vi "PM5000_Power_demo.vi"(2 "error in (no error)":errorcluster) -> (0 "error out":errorcluster, 1 "Power Meter Out":T1)   [LabVIEW 2018]
panel:
  in  "Variacion Pontencia":sgl=0.1
  in  "Potencia Nominal":sgl=20.0
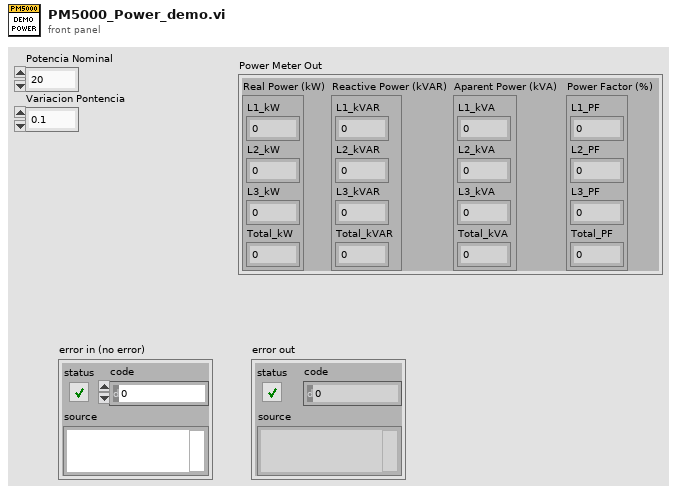
[diagram p1: front panel]
types:
  T1 = cluster{"Real Power (kW)":cluster{"L1_kW":sgl, "L2_kW":sgl, "L3_kW":sgl, "Total_kW":sgl}, "Reactive Power (kVAR)":cluster{"L1_kVAR":sgl, "L2_kVAR":sgl, "L3_kVAR":sgl, "Total_kVAR":sgl}, "Aparent Power (kVA)":cluster{"L1_kVA":sgl, "L2_kVA":sgl, "L3_kVA":sgl, "Total_kVA":sgl}, "Power Factor (%)":cluster{"L1_PF":sgl, "L2_PF":sgl, "L3_PF":sgl, "Total_PF":sgl}}
  T2 = cluster{"Real Power (kW)":cluster{"L1_kW":sgl, "L2_kW":sgl, "L3_kW":sgl, "Total_kW":sgl}, "Reactive Power (kVAR)":cluster{"L1_kVAR":sgl, "L2_kVAR":sgl, "L3_kVAR":sgl, "Total_kVAR":sgl}, "Aparent Power (kVA)":cluster{"L1_kVA":sgl, "L2_kVA":sgl, "L3_kVA":sgl, "Total_kVA":sgl}, "Power Factor":cluster{"L1_PF":sgl, "L2_PF":sgl, "L3_PF":sgl, "Total_PF":sgl}}
  T3 = cluster{"L1_PF":sgl, "L2_PF":sgl, "L3_PF":sgl, "Total_PF":sgl}
  T4 = cluster{"L1_kVA":sgl, "L2_kVA":sgl, "L3_kVA":sgl, "Total_kVA":sgl}
  T5 = cluster{"L1_kVAR":sgl, "L2_kVAR":sgl, "L3_kVAR":sgl, "Total_kVAR":sgl}
  T6 = cluster{"L1_kW":sgl, "L2_kW":sgl, "L3_kW":sgl, "Total_kW":sgl}
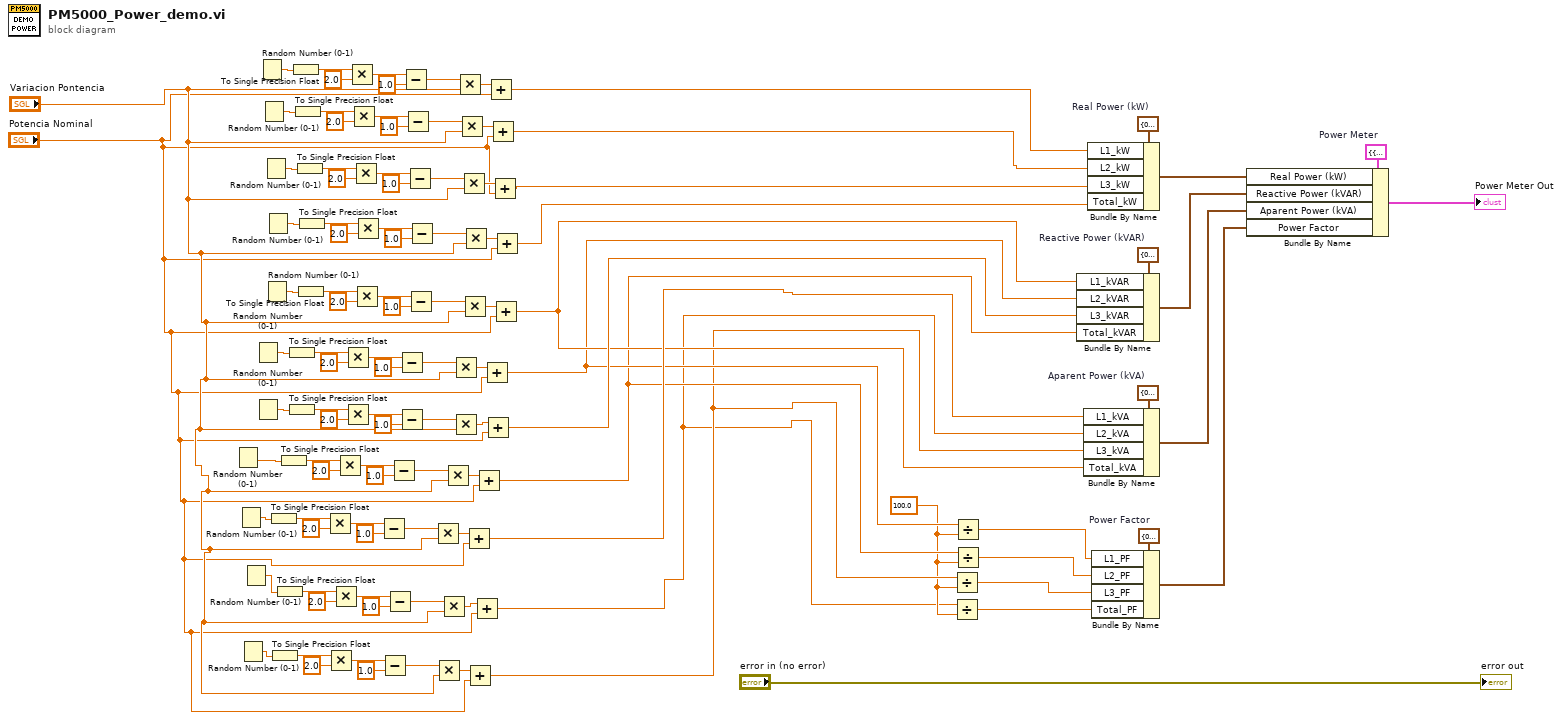
[diagram p0: block diagram]
diagram:
  w3 = sgl 100.0
  w101 = T2 {"Real Power (kW)"={"L1_kW"=-0.009145112, "L2_kW"=-0.0037322815, "L3_kW"=-0.019452685, "Total_kW"=-0.03233008}, "Reactive Power (kVAR)"={"L1_kVAR"=-0.01587091, "L2_kVAR"=-0.0369946, "L3_kVAR"=-0.038295496, "Total_kVAR"=-0.091161005}, "Aparent Power (kVA)"={"L1_kVA"=0.018485848, "L2_kVA"=0.037469197, "L3_kVA"=0.04338286, "Total_kVA"=0.099337906}, "Power Factor"={"L1_PF"=49.470882, "L2_PF"=9.960934, "L3_PF"=44.839565, "Total_PF"=32.545567}}  # Power Meter
  w102 = T3 {"L1_PF"=0.0, "L2_PF"=0.0, "L3_PF"=0.0, "Total_PF"=0.0}  # Power Factor
  w103 = T4 {"L1_kVA"=0.0, "L2_kVA"=0.0, "L3_kVA"=0.0, "Total_kVA"=0.0}  # Aparent Power (kVA)
  w104 = T5 {"L1_kVAR"=0.0, "L2_kVAR"=0.0, "L3_kVAR"=0.0, "Total_kVAR"=0.0}  # Reactive Power (kVAR)
  w105 = T6 {"L1_kW"=0.0, "L2_kW"=0.0, "L3_kW"=0.0, "Total_kW"=0.0}  # Real Power (kW)
  n1 = Random Number (0-1)() -> (number: 0 to 1=w42:dbl)
  n2 = Random Number (0-1)() -> (number: 0 to 1=w35:dbl)
  n3 = Random Number (0-1)() -> (number: 0 to 1=w21:dbl)
  n4 = Random Number (0-1)() -> (number: 0 to 1=w28:dbl)
  n5 = Random Number (0-1)() -> (number: 0 to 1=w56:dbl)
  n6 = Random Number (0-1)() -> (number: 0 to 1=w49:dbl)
  n7 = Random Number (0-1)() -> (number: 0 to 1=w92:dbl)
  n8 = Random Number (0-1)() -> (number: 0 to 1=w84:dbl)
  n9 = Random Number (0-1)() -> (number: 0 to 1=w77:dbl)
  n10 = Random Number (0-1)() -> (number: 0 to 1=w63:dbl)
  n11 = Random Number (0-1)() -> (number: 0 to 1=w70:dbl)
  n12 = To Single Precision Float(number=w35) -> (single precision float=w34:sgl)
  n13 = To Single Precision Float(number=w21) -> (single precision float=w20:sgl)
  n14 = To Single Precision Float(number=w28) -> (single precision float=w29:sgl)
  n15 = To Single Precision Float(number=w42) -> (single precision float=w43:sgl)
  n16 = To Single Precision Float(number=w56) -> (single precision float=w57:sgl)
  n17 = To Single Precision Float(number=w49) -> (single precision float=w48:sgl)
  n18 = To Single Precision Float(number=w92) -> (single precision float=w91:sgl)
  n19 = To Single Precision Float(number=w84) -> (single precision float=w85:sgl)
  n20 = To Single Precision Float(number=w77) -> (single precision float=w76:sgl)
  n21 = To Single Precision Float(number=w63) -> (single precision float=w62:sgl)
  n22 = To Single Precision Float(number=w70) -> (single precision float=w71:sgl)
  n23 = Multiply(x=w34, y=sgl 2.0) -> (x*y=w37:sgl)
  n24 = Multiply(x=w20, y=sgl 2.0) -> (x*y=w23:sgl)
  n25 = Multiply(x=w29, y=sgl 2.0) -> (x*y=w26:sgl)
  n26 = Multiply(x=w43, y=sgl 2.0) -> (x*y=w40:sgl)
  n27 = Multiply(x=w57, y=sgl 2.0) -> (x*y=w54:sgl)
  n28 = Multiply(x=w48, y=sgl 2.0) -> (x*y=w51:sgl)
  n29 = Multiply(x=w91, y=sgl 2.0) -> (x*y=w94:sgl)
  n30 = Multiply(x=w85, y=sgl 2.0) -> (x*y=w82:sgl)
  n31 = Multiply(x=w76, y=sgl 2.0) -> (x*y=w79:sgl)
  n32 = Multiply(x=w62, y=sgl 2.0) -> (x*y=w65:sgl)
  n33 = Multiply(x=w71, y=sgl 2.0) -> (x*y=w68:sgl)
  n34 = Subtract(x=w37, y=sgl 1.0) -> (x-y=w33:sgl)
  n35 = Subtract(x=w23, y=sgl 1.0) -> (x-y=w19:sgl)
  n36 = Subtract(x=w26, y=sgl 1.0) -> (x-y=w30:sgl)
  n37 = Subtract(x=w40, y=sgl 1.0) -> (x-y=w44:sgl)
  n38 = Subtract(x=w54, y=sgl 1.0) -> (x-y=w58:sgl)
  n39 = Subtract(x=w51, y=sgl 1.0) -> (x-y=w47:sgl)
  n40 = Subtract(x=w94, y=sgl 1.0) -> (x-y=w90:sgl)
  n41 = Subtract(x=w82, y=sgl 1.0) -> (x-y=w86:sgl)
  n42 = Subtract(x=w79, y=sgl 1.0) -> (x-y=w75:sgl)
  n43 = Subtract(x=w65, y=sgl 1.0) -> (x-y=w61:sgl)
  n44 = Subtract(x=w68, y=sgl 1.0) -> (x-y=w72:sgl)
  n45 = Multiply(x=w33, y="Variacion Pontencia") -> (x*y=w32:sgl)
  n46 = Multiply(x=w19, y="Variacion Pontencia") -> (x*y=w18:sgl)
  n47 = Multiply(x=w30, y="Variacion Pontencia") -> (x*y=w31:sgl)
  n48 = Multiply(x=w44, y="Variacion Pontencia") -> (x*y=w45:sgl)
  n49 = Multiply(x=w58, y="Variacion Pontencia") -> (x*y=w59:sgl)
  n50 = Multiply(x=w47, y="Variacion Pontencia") -> (x*y=w46:sgl)
  n51 = Multiply(x=w90, y="Variacion Pontencia") -> (x*y=w89:sgl)
  n52 = Multiply(x=w86, y="Variacion Pontencia") -> (x*y=w87:sgl)
  n53 = Multiply(x=w75, y="Variacion Pontencia") -> (x*y=w74:sgl)
  n54 = Multiply(x=w61, y="Variacion Pontencia") -> (x*y=w60:sgl)
  n55 = Multiply(x=w72, y="Variacion Pontencia") -> (x*y=w73:sgl)
  n56 = Add(x=w32, y="Potencia Nominal") -> (x+y=w11:sgl)
  n57 = Add(x=w18, y="Potencia Nominal") -> (x+y=w5:sgl)
  n58 = Add(x=w31, y="Potencia Nominal") -> (x+y=w2:sgl)
  n59 = Add(x=w45, y="Potencia Nominal") -> (x+y=w7:sgl)
  n60 = Add(x=w59, y="Potencia Nominal") -> (x+y=w9:sgl)
  n61 = Add(x=w46, y="Potencia Nominal") -> (x+y=w12:sgl)
  n62 = Add(x=w89, y="Potencia Nominal") -> (x+y=w88:sgl)
  n63 = Add(x=w87, y="Potencia Nominal") -> (x+y=w15:sgl)
  n64 = Add(x=w74, y="Potencia Nominal") -> (x+y=w14:sgl)
  n65 = Add(x=w60, y="Potencia Nominal") -> (x+y=w10:sgl)
  n66 = Add(x=w73, y="Potencia Nominal") -> (x+y=w13:sgl)
  n67 = Divide(x=w5, y=w3) -> (x/y=w4:sgl)
  n68 = Divide(x=w2, y=w3) -> (x/y=w1:sgl)
  n69 = Divide(x=w9, y=w3) -> (x/y=w8:sgl)
  n70 = Divide(x=w7, y=w3) -> (x/y=w6:sgl)
  n71 = Bundle By Name(cluster=w104, "L1_kVAR"=w10, "L2_kVAR"=w9, "L3_kVAR"=w12, "Total_kVAR"=w7) -> (w99:T5)
  n72 = Bundle By Name(cluster=w103, "L1_kVA"=w11, "L2_kVA"=w2, "L3_kVA"=w5, "Total_kVA"=w10) -> (w98:T4)
  n73 = Bundle By Name(cluster=w105, "L1_kW"=w88, "L2_kW"=w15, "L3_kW"=w14, "Total_kW"=w13) -> (w100:T6)
  n74 = Bundle By Name(cluster=w102, "L1_PF"=w8, "L2_PF"=w6, "L3_PF"=w4, "Total_PF"=w1) -> (w97:T3)
  n75 = Bundle By Name(cluster=w101, "Real Power (kW)"=w100, "Reactive Power (kVAR)"=w99, "Aparent Power (kVA)"=w98, "Power Factor"=w97) -> (→"Power Meter Out":T2)
  "error out" <- "error in (no error)"
